vi "Remove Corners.vi"(4 "Old Corners Matrix":i8[][](array[numeric]), 5 "Old corners":cluster{"Col":i16, "Row":i16}[](array[cluster]), 6 "Updated Map":i8[][](array[numeric])) -> (1 "Updated Corners Matrix":i8[][](array[numeric]), 2 "New old corners":cluster{"Col":i16, "Row":i16}[](array[cluster]))   [LabVIEW 2009]
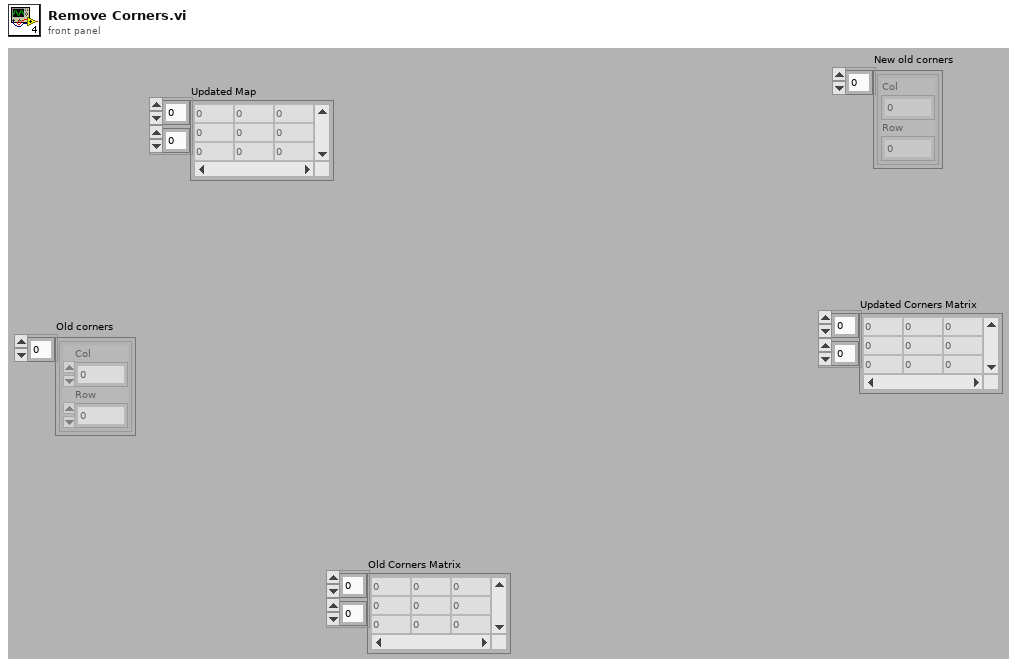
[diagram p1: front panel]
types:
  T1 = typedef "NI_Matrix.lvlib/RealMatrix.ctl" = dbl[][]
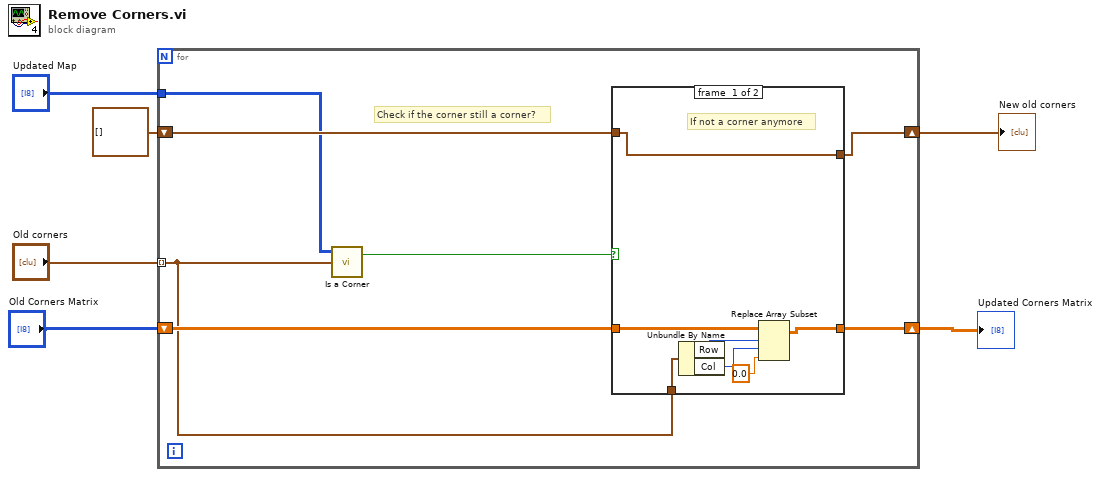
[diagram p0: block diagram]
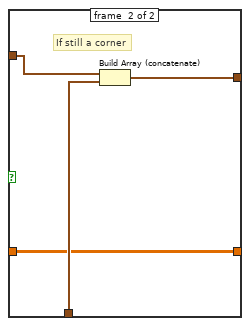
[diagram p2: hidden frame]
diagram:
  n1 = for {
    tunnel: "Old corners" -> [w7] mode=indexing
    tunnel: "Updated Map" -> [w11]
    shift-right: [w12] -> w4
    shift-left: cluster{"X":dbl, "Y":dbl}[] [] -> [w13]
    shift-right: [w8] -> w1
    shift-left: "Old Corners Matrix" -> [w9]
    # "Check if the corner still a corner?"
    n2 = call "Is a Corner.vi"("Corner candidate"=w7, "Updated Map"=w11) -> ("Is a corner"=w10:bool)  [unwired: 2 in]
    n3 = case shown="False" w10 {
      tunnel: w13 -> [w20 w24]
      tunnel: [w20 w23] -> w12
      tunnel: w7 -> [w14 w22]
      tunnel: w9 -> [w18 w21]
      tunnel: [w17 w21] -> w8
      frame #0 {
        # "If not a corner anymore"
        n4 = Unbundle By Name(w14) -> ("Row"=w16:i16, "Col"=w15:i16)
        n5 = Replace Array Subset(array=w18, new element=0.0 ("new element/submatrix"), index (row)=w16, index (col)=w15) -> (w17:T1)
      }
      frame #1 {
        # "If still a corner"
        n6 = Build Array (concatenate)(w24, w22) -> (w23:cluster{"X":dbl, "Y":dbl}[])
      }
    }
  }
  "New old corners" <- w4
  "Updated Corners Matrix" <- w1
